vi "Lift Wrapper.vi"(0 "Up or Down":bool) -> ()   [LabVIEW 2014]
uses:
  Precreated VIs/Robot Global Data.vi
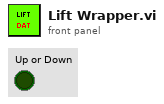
[diagram p1: front panel]
types:
  T1 = cluster{"Limit Switches":cluster{"Lift":cluster{"Lift Top":bool, "Lift High":bool, "Lift Medium":bool, "Lift Low":bool, "Lift Bottom":bool}, "Clamp":cluster{"Clamp Widest":bool, "Clamp Shortest":bool, "Tote Left":bool, "Tote Right":bool}}, "Ultrasonic":dbl, "Arm Beam Breaker":bool, "Tote Beam Breaker":bool, "Lift Encoder":cluster{"Distance":dbl, "Rate":dbl, "Direction":bool, "Stopped":bool}, "Drive Encoders":cluster{"Distance":dbl, "Rate":dbl, "Direction":bool, "Stopped":bool}[]}
  T2 = cluster{"Lift Top":bool, "Lift High":bool, "Lift Medium":bool, "Lift Low":bool, "Lift Bottom":bool}
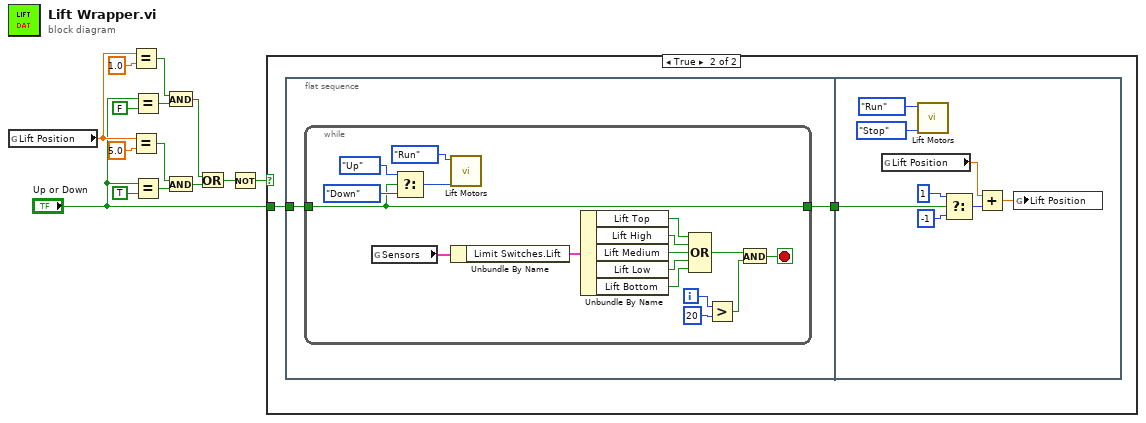
[diagram p0: block diagram]
diagram:
  n1 = global read "Robot Global Data.vi" "Lift Position"() -> (w11:dbl)
  n2 = Equal?(x=w11, y=1.0) -> (x = y?=w9:bool)
  n3 = Equal?(x=w11, y=5.0) -> (x = y?=w6:bool)
  n4 = Equal?(x="Up or Down", y=FALSE) -> (x = y?=w12:bool)
  n5 = Equal?(x="Up or Down", y=TRUE) -> (x = y?=w7:bool)
  n6 = And(x=w9, y=w12) -> (x .and. y?=w5:bool)
  n7 = And(x=w6, y=w7) -> (x .and. y?=w4:bool)
  n8 = Or(x=w5, y=w4) -> (x .or. y?=w3:bool)
  n9 = Not(x=w3) -> (.not. x?=w2:bool)
  n10 = case shown="True" w2 {
    tunnel: "Up or Down" -> [_ w16]
    frame False {
    }
    frame True {
      n11 = flat-sequence {
        tunnel: w16 -> [w18]
        tunnel: [w17] -> w15
        tunnel: w15 -> [w36]
        frame #0 {
          n12 = while {
            tunnel: w18 -> [w19]
            tunnel: [w19] -> w17
            i -> [w35]
            stop <- w23 stop-if-true
            n13 = global read "Robot Global Data.vi" "Sensors"() -> (w21:T1)
            n14 = Select(t=enum16{"Stop", "Up", "Down"}."Up" ("Direction"), s=w19, f=enum16{"Stop", "Up", "Down"}."Down" ("Direction")) -> (s? t:f=w32:enum16{"Stop", "Up", "Down"})
            n15 = call "Lift Motors.vi"("Direction"=w32, "Mode"=enum8{"Start", "Run", "Finish"}."Run") -> ()  [unwired: 2 in]
            n16 = Unbundle By Name(w21) -> ("Limit Switches.Lift"=w20:T2)
            n17 = Unbundle By Name(w20) -> ("Lift Top"=w27:bool, "Lift High"=w28:bool, "Lift Medium"=w29:bool, "Lift Low"=w30:bool, "Lift Bottom"=w31:bool)
            n18 = Compound Arithmetic op=OR(w27, w28, w29, w30, w31) -> (w25:bool)
            n19 = Greater?(x=w35, y=20) -> (0:w24:bool)
            n20 = And(x=w25, y=w24) -> (x .and. y?=w23:bool)
          }
        }
        frame #1 {
          n21 = global read "Robot Global Data.vi" "Lift Position"() -> (w43:dbl)
          n22 = call "Lift Motors.vi"("Direction"=enum16{"Stop", "Up", "Down"}."Stop", "Mode"=enum8{"Start", "Run", "Finish"}."Run") -> ()  [unwired: 2 in]
          n23 = Select(t=1, s=w36, f=-1) -> (s? t:f=w40:i32)
          n24 = Add(x=w43, y=w40) -> (x+y=w42:dbl)
          n25 = global write "Robot Global Data.vi" "Lift Position"(w42) -> ()
        }
      }
    }
  }
